vi "Gen_UV_CMD (SubVI).vi"(1 "value":string, 2 "function":string) -> (0 "commu_data":string)   [LabVIEW 2014]
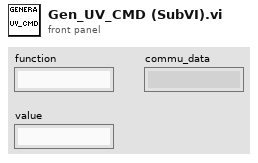
[diagram p1: front panel]
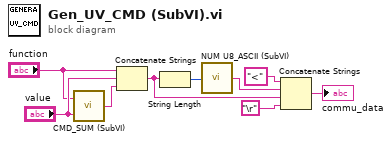
[diagram p0: block diagram]
diagram:
  n1 = call "CMD_SUM (SubVI).vi"("value"="value", "Func"="function") -> ("String"=w7:string)
  n2 = Concatenate Strings("function", "value", w7) -> (w4:string)
  n3 = String Length(string=w4) -> (length=w1:i32)
  n4 = call "NUM U8_ASCII (SubVI).vi"("Numeric"=w1) -> ("String out"=w3:string)
  n5 = Concatenate Strings("<", w3, w4, "\r") -> (→"commu_data":string)
